vi "GeoData.vi"() -> ()   [LabVIEW 2017] (continued)
MN\tTodd County\tH1\n56331\t27153\tFreeport\tMN\tTodd County\tH1\n56378\t27153\tSauk centre\tMN\tTodd County\tH1\n56318\t27153\tBurtrum\tMN\tTodd County\tH1\n56440\t27153\tClarissa\tMN\tTodd County\tH1\n56482\t27153\tWadena\tMN\tTodd County\tH1\n56466\t27153\tMotley\tMN\tTodd County\tH1\n56446\t27153\tEagle bend\tMN\tTodd County\tH1\n56475\t27153\tRandall\tMN\tTodd County\tH1\n56389\t27153\tWest union\tMN\tTodd County\tH1\n56434\t27153\tAldrich\tMN\tTodd County\tH1\n56382\t27153\tSwanville\tMN\tTodd County\tH1\n56219\t27155\tBrowns valley\tMN\tTraverse County\tH1\n56236\t27155\tDumont\tMN\tTraverse County\tH1\n56274\t27155\tNorcross\tMN\tTraverse County\tH1\n56565\t27155\tNashua\tMN\tTraverse County\tH1\n56296\t27155\tWheaton\tMN\tTraverse County\tH1\n56211\t27155\tBeardsley\tMN\tTraverse County\tH1\n56248\t27155\tHerman\tMN\tTraverse County\tH1\n56240\t27155\tGraceville\tMN\tTraverse County\tH1\n56583\t27155\tTintah\tMN\tTraverse County\tH1\n56522\t27155\tCampbell\tMN\tTraverse County\tH1\n56221\t27155\tChokio\tMN\tTraverse County\tH1\n55906\t27157\tRochester\tMN\tWabasha County\tH1\n55960\t27157\tOronoco\tMN\tWabasha County\tH1\n55957\t27157\tMillville\tMN\tWabasha County\tH1\n55041\t27157\tLake city\tMN\tWabasha County\tH1\n55991\t27157\tZumbro falls\tMN\tWabasha County\tH1\n55027\t27157\tGoodhue\tMN\tWabasha County\tH1\n55932\t27157\tElgin\tMN\tWabasha County\tH1\n55956\t27157\tMazeppa\tMN\tWabasha County\tH1\n55910\t27157\tAltura\tMN\tWabasha County\tH1\n55945\t27157\tKellogg\tMN\tWabasha County\tH1\n55964\t27157\tPlainview\tMN\tWabasha County\tH1\n55968\t27157\tReads landing\tMN\tWabasha County\tH1\n55981\t27157\tWabasha\tMN\tWabasha County\tH1\n56481\t27159\tVerndale\tMN\tWadena County\tH1\n56464\t27159\tMenahga\tMN\tWadena County\tH1\n56470\t27159\tPark rapids\tMN\tWadena County\tH1\n56479\t27159\tStaples\tMN\tWadena County\tH1\n56477\t27159\tSebeka\tMN\tWadena County\tH1\n56482\t27159\tWadena\tMN\tWadena County\tH1\n56434\t27159\tAldrich\tMN\tWadena County\tH1\n56096\t27161\tWaterville\tMN\tWaseca County\tH1\n56068\t27161\tMinnesota lake\tMN\tWaseca County\tH1\n56078\t27161\tPemberton\tMN\tWaseca County\tH1\n56091\t27161\tWaldorf\tMN\tWaseca County\tH1\n56026\t27161\tEllendale\tMN\tWaseca County\tH1\n56063\t27161\tMadison lake\tMN\tWaseca County\tH1\n56093\t27161\tWaseca\tMN\tWaseca County\tH1\n56072\t27161\tNew richland\tMN\tWaseca County\tH1\n56042\t27161\tHartland\tMN\tWaseca County\tH1\n56065\t27161\tMapleton\tMN\tWaseca County\tH1\n56028\t27161\tElysian\tMN\tWaseca County\tH1\n56048\t27161\tJanesville\tMN\tWaseca County\tH1\n56097\t27161\tWells\tMN\tWaseca County\tH1\n55052\t27161\tMorristown\tMN\tWaseca County\tH1\n55071\t27163\tSaint paul park\tMN\tWashington County\tH1\n55016\t27163\tCottage grove\tMN\tWashington County\tH1\n55001\t27163\tAfton\tMN\tWashington County\tH1\n55042\t27163\tLake elmo\tMN\tWashington County\tH1\n55033\t27163\tHastings\tMN\tWashington County\tH1\n55013\t27163\tChisago city\tMN\tWashington County\tH1\n55043\t27163\tLakeland\tMN\tWashington County\tH1\n55055\t27163\tNewport\tMN\tWashington County\tH1\n55047\t27163\tMarine on saint croix\tMN\tWashington County\tH1\n55119\t27163\tSaint paul\tMN\tWashington County\tH1\n55025\t27163\tForest lake\tMN\tWashington County\tH1\n55073\t27163\tScandia\tMN\tWashington County\tH1\n55109\t27163\tSaint paul\tMN\tWashington County\tH1\n55125\t27163\tSaint paul\tMN\tWashington County\tH1\n55038\t27163\tHugo\tMN\tWashington County\tH1\n55082\t27163\tStillwater\tMN\tWashington County\tH1\n55115\t27163\tSaint paul\tMN\tWashington County\tH1\n55083\t27163\tStillwater\tMN\tWashington County\tH1\n55003\t27163\tBayport\tMN\tWashington County\tH1\n55110\t27163\tSaint paul\tMN\tWashington County\tH1\n55128\t27163\tSaint paul\tMN\tWashington County\tH1\n55129\t27163\tSaint paul\tMN\tWashington County\tH1\n55090\t27163\tWillernie\tMN\tWashington County\tH1\n56159\t27165\tMountain lake\tMN\tWatonwan County\tH1\n56162\t27165\tOrmsby\tMN\tWatonwan County\tH1\n56160\t27165\tOdin\tMN\tWatonwan County\tH1\n56081\t27165\tSaint james\tMN\tWatonwan County\tH1\n56022\t27165\tDarfur\tMN\tWatonwan County\tH1\n56056\t27165\tLa salle\tMN\tWatonwan County\tH1\n56062\t27165\tMadelia\tMN\tWatonwan County\tH1\n56041\t27165\tHanska\tMN\tWatonwan County\tH1\n56019\t27165\tComfrey\tMN\tWatonwan County\tH1\n56120\t27165\tButterfield\tMN\tWatonwan County\tH1\n56060\t27165\tLewisville\tMN\tWatonwan County\tH1\n56088\t27165\tTruman\tMN\tWatonwan County\tH1\n56565\t27167\tNashua\tMN\tWilkin County\tH1\n56520\t27167\tBreckenridge\tMN\tWilkin County\tH1\n56594\t27167\tWolverton\tMN\tWilkin County\tH1\n56543\t27167\tFoxhome\tMN\tWilkin County\tH1\n56579\t27167\tRothsay\tMN\tWilkin County\tH1\n56583\t27167\tTintah\tMN\tWilkin County\tH1\n56522\t27167\tCampbell\tMN\tWilkin County\tH1\n56514\t27167\tBarnesville\tMN\tWilkin County\tH1\n56572\t27167\tPelican rapids\tMN\tWilkin County\tH1\n56553\t27167\tKent\tMN\tWilkin County\tH1\n55952\t27169\tLewiston\tMN\tWinona County\tH1\n55987\t27169\tWinona\tMN\tWinona County\tH1\n55923\t27169\tChatfield\tMN\tWinona County\tH1\n55959\t27169\tMinnesota city\tMN\tWinona County\tH1\n55971\t27169\tRushford\tMN\tWinona County\tH1\n55962\t27169\tPeterson\tMN\tWinona County\tH1\n55972\t27169\tSaint charles\tMN\tWinona County\tH1\n55979\t27169\tUtica\tMN\tWinona County\tH1\n55947\t27169\tLa crescent\tMN\tWinona County\tH1\n55969\t27169\tRollingstone\tMN\tWinona County\tH1\n55910\t27169\tAltura\tMN\tWinona County\tH1\n55943\t27169\tHouston\tMN\tWinona County\tH1\n55964\t27169\tPlainview\tMN\tWinona County\tH1\n55925\t27169\tDakota\tMN\tWinona County\tH1\n55363\t27171\tMontrose\tMN\tWright County\tH1\n55341\t27171\tHanover\tMN\tWright County\tH1\n55327\t27171\tDayton\tMN\tWright County\tH1\n55376\t27171\tSaint michael\tMN\tWright County\tH1\n55330\t27171\tElk river\tMN\tWright County\tH1\n55313\t27171\tBuffalo\tMN\tWright County\tH1\n55321\t27171\tCokato\tMN\tWright County\tH1\n55328\t27171\tDelano\tMN\tWright County\tH1\n55362\t27171\tMonticello\tMN\tWright County\tH1\n55373\t27171\tRockford\tMN\tWright County\tH1\n55388\t27171\tWatertown\tMN\tWright County\tH1\n55358\t27171\tMaple lake\tMN\tWright County\tH1\n55382\t27171\tSouth haven\tMN\tWright County\tH1\n55381\t27171\tSilver lake\tMN\tWright County\tH1\n55374\t27171\tRogers\tMN\tWright County\tH1\n55301\t27171\tAlbertville\tMN\tWright County\tH1\n55320\t27171\tClearwater\tMN\tWright County\tH1\n55302\t27171\tAnnandale\tMN\tWright County\tH1\n55390\t27171\tWaverly\tMN\tWright County\tH1\n55349\t27171\tHoward lake\tMN\tWright County\tH1\n55325\t27171\tDassel\tMN\tWright County\tH1\n55395\t27171\tWinsted\tMN\tWright County\tH1\n56264\t27173\tMinneota\tMN\tYellow Medicine County\tH1\n56223\t27173\tClarkfield\tMN\tYellow Medicine County\tH1\n56291\t27173\tTaunton\tMN\tYellow Medicine County\tH1\n56256\t27173\tMadison\tMN\tYellow Medicine County\tH1\n56241\t27173\tGranite falls\tMN\tYellow Medicine County\tH1\n56142\t27173\tIvanhoe\tMN\tYellow Medicine County\tH1\n56220\t27173\tCanby\tMN\tYellow Medicine County\tH1\n56265\t27173\tMontevideo\tMN\tYellow Medicine County\tH1\n56292\t27173\tVesta\tMN\tYellow Medicine County\tH1\n56214\t27173\tBelview\tMN\tYellow Medicine County\tH1\n56297\t27173\tWood lake\tMN\tYellow Medicine County\tH1\n56218\t27173\tBoyd\tMN\tYellow Medicine County\tH1\n56229\t27173\tCottonwood\tMN\tYellow Medicine County\tH1\n56237\t27173\tEcho\tMN\tYellow Medicine County\tH1\n56245\t27173\tHanley falls\tMN\tYellow Medicine County\tH1\n56280\t27173\tPorter\tMN\tYellow Medicine County\tH1\n39121\t28001\tNatchez\tMS\tAdams County\tH1\n39661\t28001\tRoxie\tMS\tAdams County\tH1\n39122\t28001\tNatchez\tMS\tAdams County\tH1\n39190\t28001\tWashington\tMS\tAdams County\tH1\n39165\t28001\tSibley\tMS\tAdams County\tH1\n39120\t28001\tNatchez\tMS\tAdams County\tH1\n38846\t28003\tGlen\tMS\tAlcorn County\tH1\n38683\t28003\tWalnut\tMS\tAlcorn County\tH1\n38833\t28003\tBurnsville\tMS\tAlcorn County\tH1\n38865\t28003\tRienzi\tMS\tAlcorn County\tH1\n38835\t28003\tCorinth\tMS\tAlcorn County\tH1\n38834\t28003\tCorinth\tMS\tAlcorn County\tH1\n39638\t28005\tGloster\tMS\tAmite County\tH1\n39652\t28005\tMagnolia\tMS\tAmite County\tH1\n39633\t28005\tCrosby\tMS\tAmite County\tH1\n39645\t28005\tLiberty\tMS\tAmite County\tH1\n39631\t28005\tCentreville\tMS\tAmite County\tH1\n39666\t28005\tSummit\tMS\tAmite County\tH1\n39657\t28005\tOsyka\tMS\tAmite County\tH1\n39664\t28005\tSmithdale\tMS\tAmite County\tH1\n39653\t28005\tMeadville\tMS\tAmite County\tH1\n39051\t28007\tCarthage\tMS\tAttala County\tH1\n39192\t28007\tWest\tMS\tAttala County\tH1\n39090\t28007\tKosciusko\tMS\tAttala County\tH1\n39079\t28007\tGoodman\tMS\tAttala County\tH1\n39772\t28007\tWeir\tMS\tAttala County\tH1\n39108\t28007\tMc cool\tMS\tAttala County\tH1\n39160\t28007\tSallis\tMS\tAttala County\tH1\n39067\t28007\tEthel\tMS\tAttala County\tH1\n39176\t28007\tVaiden\tMS\tAttala County\tH1\n38635\t28009\tHolly springs\tMS\tBenton County\tH1\n38603\t28009\tAshland\tMS\tBenton County\tH1\n38629\t28009\tFalkner\tMS\tBenton County\tH1\n38683\t28009\tWalnut\tMS\tBenton County\tH1\n38650\t28009\tMyrtle\tMS\tBenton County\tH1\n38610\t28009\tBlue mountain\tMS\tBenton County\tH1\n38633\t28009\tHickory flat\tMS\tBenton County\tH1\n38647\t28009\tMichigan city\tMS\tBenton County\tH1\n38642\t28009\tLamar\tMS\tBenton County\tH1\n38663\t28009\tRipley\tMS\tBenton County\tH1\n38659\t28009\tPotts camp\tMS\tBenton County\tH1\n38769\t28011\tRosedale\tMS\tBolivar County\tH1\n38746\t28011\tGunnison\tMS\tBolivar County\tH1\n38781\t28011\tWinstonville\tMS\tBolivar County\tH1\n38733\t28011\tCleveland\tMS\tBolivar County\tH1\n38762\t28011\tMound bayou\tMS\tBolivar County\tH1\n38720\t28011\tAlligator\tMS\tBolivar County\tH1\n38764\t28011\tPace\tMS\tBolivar County\tH1\n38740\t28011\tDuncan\tMS\tBolivar County\tH1\n38772\t28011\tScott\tMS\tBolivar County\tH1\n38726\t28011\tBeulah\tMS\tBolivar County\tH1\n38759\t28011\tMerigold\tMS\tBolivar County\tH1\n38774\t28011\tShelby\tMS\tBolivar County\tH1\n38730\t28011\tBoyle\tMS\tBolivar County\tH1\n38614\t28011\tClarksdale\tMS\tBolivar County\tH1\n38732\t28011\tCleveland\tMS\tBolivar County\tH1\n38703\t28011\tGreenville\tMS\tBolivar County\tH1\n38725\t28011\tBenoit\tMS\tBolivar County\tH1\n38773\t28011\tShaw\tMS\tBolivar County\tH1\n38951\t28013\tPittsboro\tMS\tCalhoun County\tH1\n38929\t28013\tGore springs\tMS\tCalhoun County\tH1\n38839\t28013\tDerma\tMS\tCalhoun County\tH1\n38851\t28013\tHouston\tMS\tCalhoun County\tH1\n38913\t28013\tBanner\tMS\tCalhoun County\tH1\n38850\t28013\tHoulka\tMS\tCalhoun County\tH1\n38864\t28013\tRandolph\tMS\tCalhoun County\tH1\n38915\t28013\tBruce\tMS\tCalhoun County\tH1\n38878\t28013\tVardaman\tMS\tCalhoun County\tH1\n38914\t28013\tBig creek\tMS\tCalhoun County\tH1\n38916\t28013\tCalhoun city\tMS\tCalhoun County\tH1\n38965\t28013\tWater valley\tMS\tCalhoun County\tH1\n38954\t28015\tSidon\tMS\tCarroll County\tH1\n39192\t28015\tWest\tMS\tCarroll County\tH1\n38943\t28015\tMc carley\tMS\tCarroll County\tH1\n38947\t28015\tNorth carrollton\tMS\tCarroll County\tH1\n38917\t28015\tCarrollton\tMS\tCarroll County\tH1\n38924\t28015\tCruger\tMS\tCarroll County\tH1\n38930\t28015\tGreenwood\tMS\tCarroll County\tH1\n38967\t28015\tWinona\tMS\tCarroll County\tH1\n38940\t28015\tHolcomb\tMS\tCarroll County\tH1\n38923\t28015\tCoila\tMS\tCarroll County\tH1\n39176\t28015\tVaiden\tMS\tCarroll County\tH1\n38868\t28017\tShannon\tMS\tChickasaw County\tH1\n38851\t28017\tHouston\tMS\tChickasaw County\tH1\n38877\t28017\tVan vleet\tMS\tChickasaw County\tH1\n38850\t28017\tHoulka\tMS\tChickasaw County\tH1\n38860\t28017\tOkolona\tMS\tChickasaw County\tH1\n38878\t28017\tVardaman\tMS\tChickasaw County\tH1\n39756\t28017\tPrairie\tMS\tChickasaw County\tH1\n39730\t28017\tAberdeen\tMS\tChickasaw County\tH1\n39751\t28017\tMantee\tMS\tChickasaw County\tH1\n39776\t28017\tWoodland\tMS\tChickasaw County\tH1\n38875\t28017\tTrebloc\tMS\tChickasaw County\tH1\n39752\t28019\tMathiston\tMS\tChoctaw County\tH1\n39744\t28019\tEupora\tMS\tChoctaw County\tH1\n39767\t28019\tStewart\tMS\tChoctaw County\tH1\n39772\t28019\tWeir\tMS\tChoctaw County\tH1\n39108\t28019\tMc cool\tMS\tChoctaw County\tH1\n39745\t28019\tFrench camp\tMS\tChoctaw County\tH1\n39750\t28019\tMaben\tMS\tChoctaw County\tH1\n39735\t28019\tAckerman\tMS\tChoctaw County\tH1\n39769\t28019\tSturgis\tMS\tChoctaw County\tH1\n39144\t28021\tPattison\tMS\tClaiborne County\tH1\n39096\t28021\tLorman\tMS\tClaiborne County\tH1\n39150\t28021\tPort gibson\tMS\tClaiborne County\tH1\n39175\t28021\tUtica\tMS\tClaiborne County\tH1\n39086\t28021\tHermanville\tMS\tClaiborne County\tH1\n39363\t28023\tStonewall\tMS\tClarke County\tH1\n39307\t28023\tMeridian\tMS\tClarke County\tH1\n39360\t28023\tShubuta\tMS\tClarke County\tH1\n39367\t28023\tWaynesboro\tMS\tClarke County\tH1\n39439\t28023\tHeidelberg\tMS\tClarke County\tH1\n39355\t28023\tQuitman\tMS\tClarke County\tH1\n39366\t28023\tVossburg\tMS\tClarke County\tH1\n39347\t28023\tPachuta\tMS\tClarke County\tH1\n39301\t28023\tMeridian\tMS\tClarke County\tH1\n39330\t28023\tEnterprise\tMS\tClarke County\tH1\n39741\t28025\tCedarbluff\tMS\tClay County\tH1\n39773\t28025\tWest point\tMS\tClay County\tH1\n39755\t28025\tPheba\tMS\tClay County\tH1\n38860\t28025\tOkolona\tMS\tClay County\tH1\n39759\t28025\tStarkville\tMS\tClay County\tH1\n39756\t28025\tPrairie\tMS\tClay County\tH1\n39751\t28025\tMantee\tMS\tClay County\tH1\n39750\t28025\tMaben\tMS\tClay County\tH1\n39776\t28025\tWoodland\tMS\tClay County\tH1\n38626\t28027\tDundee\tMS\tCoahoma County\tH1\n38720\t28027\tAlligator\tMS\tCoahoma County\tH1\n38767\t28027\tRena lara\tMS\tCoahoma County\tH1\n38631\t28027\tFriars point\tMS\tCoahoma County\tH1\n38643\t28027\tLambert\tMS\tCoahoma County\tH1\n38963\t28027\tTutwiler\tMS\tCoahoma County\tH1\n38614\t28027\tClarksdale\tMS\tCoahoma County\tH1\n38617\t28027\tCoahoma\tMS\tCoahoma County\tH1\n38639\t28027\tJonestown\tMS\tCoahoma County\tH1\n38645\t28027\tLyon\tMS\tCoahoma County\tH1\n38739\t28027\tDublin\tMS\tCoahoma County\tH1\n38644\t28027\tLula\tMS\tCoahoma County\tH1\n39191\t28029\tWesson\tMS\tCopiah County\tH1\n39170\t28029\tTerry\tMS\tCopiah County\tH1\n39077\t28029\tGallman\tMS\tCopiah County\tH1\n39144\t28029\tPattison\tMS\tCopiah County\tH1\n39175\t28029\tUtica\tMS\tCopiah County\tH1\n39654\t28029\tMonticello\tMS\tCopiah County\tH1\n39083\t28029\tHazlehurst\tMS\tCopiah County\tH1\n39078\t28029\tGeorgetown\tMS\tCopiah County\tH1\n39059\t28029\tCrystal springs\tMS\tCopiah County\tH1\n39086\t28029\tHermanville\tMS\tCopiah County\tH1\n39668\t28029\tUnion church\tMS\tCopiah County\tH1\n39119\t28031\tMount olive\tMS\tCovington County\tH1\n39401\t28031\tHattiesburg\tMS\tCovington County\tH1\n39168\t28031\tTaylorsville\tMS\tCovington County\tH1\n39402\t28031\tHattiesburg\tMS\tCovington County\tH1\n39428\t28031\tCollins\tMS\tCovington County\tH1\n39479\t28031\tSeminary\tMS\tCovington County\tH1\n39474\t28031\tPrentiss\tMS\tCovington County\tH1\n39482\t28031\tSumrall\tMS\tCovington County\tH1\n39437\t28031\tEllisville\tMS\tCovington County\tH1\n38686\t28033\tWalls\tMS\tDeSoto County\tH1\n38632\t28033\tHernando\tMS\tDeSoto County\tH1\n38637\t28033\tHorn lake\tMS\tDeSoto County\tH1\n38671\t28033\tSouthaven\tMS\tDeSoto County\tH1\n38680\t28033\tWalls\tMS\tDeSoto County\tH1\n38641\t28033\tLake cormorant\tMS\tDeSoto County\tH1\n38611\t28033\tByhalia\tMS\tDeSoto County\tH1\n38618\t28033\tColdwater\tMS\tDeSoto County\tH1\n38654\t28033\tOlive branch\tMS\tDeSoto County\tH1\n38651\t28033\tNesbit\tMS\tDeSoto County\tH1\n38672\t28033\tSouthaven\tMS\tDeSoto County\tH1\n39403\t28035\tHattiesburg\tMS\tForrest County\tH1\n39465\t28035\tPetal\tMS\tForrest County\tH1\n39577\t28035\tWiggins\tMS\tForrest County\tH1\n39407\t28035\tHattiesburg\tMS\tForrest County\tH1\n39401\t28035\tHattiesburg\tMS\tForrest County\tH1\n39425\t28035\tBrooklyn\tMS\tForrest County\tH1\n39402\t28035\tHattiesburg\tMS\tForrest County\tH1\n39455\t28035\tLumberton\tMS\tForrest County\tH1\n39404\t28035\tHattiesburg\tMS\tForrest County\tH1\n39406\t28035\tHattiesburg\tMS\tForrest County\tH1\n39437\t28035\tEllisville\tMS\tForrest County\tH1\n39475\t28035\tPurvis\tMS\tForrest County\tH1\n39647\t28037\tMc call creek\tMS\tFranklin County\tH1\n39661\t28037\tRoxie\tMS\tFranklin County\tH1\n39601\t28037\tBrookhaven\tMS\tFranklin County\tH1\n39664\t28037\tSmithdale\tMS\tFranklin County\tH1\n39653\t28037\tMeadville\tMS\tFranklin County\tH1\n39668\t28037\tUnion church\tMS\tFranklin County\tH1\n39630\t28037\tBude\tMS\tFranklin County\tH1\n39456\t28039\tMc lain\tMS\tGeorge County\tH1\n39452\t28039\tLucedale\tMS\tGeorge County\tH1\n39573\t28039\tPerkinston\tMS\tGeorge County\tH1\n39456\t28041\tMc lain\tMS\tGreene County\tH1\n39362\t28041\tState line\tMS\tGreene County\tH1\n39476\t28041\tRichton\tMS\tGreene County\tH1\n39423\t28041\tBeaumont\tMS\tGreene County\tH1\n39451\t28041\tLeakesville\tMS\tGreene County\tH1\n39452\t28041\tLucedale\tMS\tGreene County\tH1\n39461\t28041\tNeely\tMS\tGreene County\tH1\n38925\t28043\tDuck hill\tMS\tGrenada County\tH1\n38929\t28043\tGore springs\tMS\tGrenada County\tH1\n39744\t28043\tEupora\tMS\tGrenada County\tH1\n38922\t28043\tCoffeeville\tMS\tGrenada County\tH1\n38920\t28043\tCascilla\tMS\tGrenada County\tH1\n38953\t28043\tScobey\tMS\tGrenada County\tH1\n38914\t28043\tBig creek\tMS\tGrenada County\tH1\n38960\t28043\tTie plant\tMS\tGrenada County\tH1\n38901\t28043\tGrenada\tMS\tGrenada County\tH1\n38940\t28043\tHolcomb\tMS\tGrenada County\tH1\n38961\t28043\tTillatoba\tMS\tGrenada County\tH1\n39556\t28045\tKiln\tMS\tHancock County\tH1\n39426\t28045\tCarriere\tMS\tHancock County\tH1\n39466\t28045\tPicayune\tMS\tHancock County\tH1\n39470\t28045\tPoplarville\tMS\tHancock County\tH1\n39520\t28045\tBay saint louis\tMS\tHancock County\tH1\n39572\t28045\tPearlington\tMS\tHancock County\tH1\n39558\t28045\tLakeshore\tMS\tHancock County\tH1\n39576\t28045\tWaveland\tMS\tHancock County\tH1\n39571\t28045\tPass christian\tMS\tHancock County\tH1\n39525\t28045\tDiamondhead\tMS\tHancock County\tH1\n39573\t28045\tPerkinston\tMS\tHancock County\tH1\n39529\t28045\tStennis space center\tMS\tHancock County\tH1\n39522\t28045\tStennis space center\tMS\tHancock County\tH1\n39560\t28047\tLong beach\tMS\tHarrison County\tH1\n39507\t28047\tGulfport\tMS\tHarrison County\tH1\n39530\t28047\tBiloxi\tMS\tHarrison County\tH1\n39501\t28047\tGulfport\tMS\tHarrison County\tH1\n39574\t28047\tSaucier\tMS\tHarrison County\tH1\n39534\t28047\tBiloxi\tMS\tHarrison County\tH1\n39565\t28047\tVancleave\tMS\tHarrison County\tH1\n39532\t28047\tBiloxi\tMS\tHarrison County\tH1\n39540\t28047\tDiberville\tMS\tHarrison County\tH1\n39535\t28047\tBiloxi\tMS\tHarrison County\tH1\n39503\t28047\tGulfport\tMS\tHarrison County\tH1\n39531\t28047\tBiloxi\tMS\tHarrison County\tH1\n39506\t28047\tGulfport\tMS\tHarrison County\tH1\n39533\t28047\tBiloxi\tMS\tHarrison County\tH1\n39571\t28047\tPass christian\tMS\tHarrison County\tH1\n39573\t28047\tPerkinston\tMS\tHarrison County\tH1\n39505\t28047\tGulfport\tMS\tHarrison County\tH1\n39502\t28047\tGulfport\tMS\tHarrison County\tH1\n39066\t28049\tEdwards\tMS\tHinds County\tH1\n39201\t28049\tJackson\tMS\tHinds County\tH1\n39205\t28049\tJackson\tMS\tHinds County\tH1\n39217\t28049\tJackson\tMS\tHinds County\tH1\n39210\t28049\tJackson\tMS\tHinds County\tH1\n39286\t28049\tJackson\tMS\tHinds County\tH1\n39211\t28049\tJackson\tMS\tHinds County\tH1\n39206\t28049\tJackson\tMS\tHinds County\tH1\n39272\t28049\tByram\tMS\tHinds County\tH1\n39170\t28049\tTerry\tMS\tHinds County\tH1\n39203\t28049\tJackson\tMS\tHinds County\tH1\n39216\t28049\tJackson\tMS\tHinds County\tH1\n39215\t28049\tJackson\tMS\tHinds County\tH1\n39283\t28049\tJackson\tMS\tHinds County\tH1\n39212\t28049\tJackson\tMS\tHinds County\tH1\n39204\t28049\tJackson\tMS\tHinds County\tH1\n39175\t28049\tUtica\tMS\tHinds County\tH1\n39207\t28049\tJackson\tMS\tHinds County\tH1\n39296\t28049\tJackson\tMS\tHinds County\tH1\n39059\t28049\tCrystal springs\tMS\tHinds County\tH1\n39060\t28049\tClinton\tMS\tHinds County\tH1\n39202\t28049\tJackson\tMS\tHinds County\tH1\n39209\t28049\tJackson\tMS\tHinds County\tH1\n39213\t28049\tJackson\tMS\tHinds County\tH1\n39058\t28049\tClinton\tMS\tHinds County\tH1\n39086\t28049\tHermanville\tMS\tHinds County\tH1\n39232\t28049\tFlowood\tMS\tHinds County\tH1\n39174\t28049\tTougaloo\tMS\tHinds County\tH1\n39269\t28049\tJackson\tMS\tHinds County\tH1\n39056\t28049\tClinton\tMS\tHinds County\tH1\n39041\t28049\tBolton\tMS\tHinds County\tH1\n39154\t28049\tRaymond\tMS\tHinds County\tH1\n39208\t28049\tPearl\tMS\tHinds County\tH1\n39236\t28049\tJackson\tMS\tHinds County\tH1\n39284\t28049\tJackson\tMS\tHinds County\tH1\n39225\t28049\tJackson\tMS\tHinds County\tH1\n38954\t28051\tSidon\tMS\tHolmes County\tH1\n39192\t28051\tWest\tMS\tHolmes County\tH1\n39146\t28051\tPickens\tMS\tHolmes County\tH1\n39038\t28051\tBelzoni\tMS\tHolmes County\tH1\n39079\t28051\tGoodman\tMS\tHolmes County\tH1\n39169\t28051\tTchula\tMS\tHolmes County\tH1\n38924\t28051\tCruger\tMS\tHolmes County\tH1\n39095\t28051\tLexington\tMS\tHolmes County\tH1\n39063\t28051\tDurant\tMS\tHolmes County\tH1\n38753\t28053\tInverness\tMS\tHumphreys County\tH1\n38754\t28053\tIsola\tMS\tHumphreys County\tH1\n39194\t28053\tYazoo city\tMS\tHumphreys County\tH1\n39115\t28053\tMidnight\tMS\tHumphreys County\tH1\n39166\t28053\tSilver city\tMS\tHumphreys County\tH1\n39038\t28053\tBelzoni\tMS\tHumphreys County\tH1\n39097\t28053\tLouise\tMS\tHumphreys County\tH1\n39159\t28055\tRolling fork\tMS\tIssaquena County\tH1\n39113\t28055\tMayersville\tMS\tIssaquena County\tH1\n39183\t28055\tVicksburg\tMS\tIssaquena County\tH1\n38744\t28055\tGlen allan\tMS\tIssaquena County\tH1\n39177\t28055\tValley park\tMS\tIssaquena County\tH1\n38745\t28055\tGrace\tMS\tIssaquena County\tH1\n38849\t28057\tGuntown\tMS\tItawamba County\tH1\n38848\t28057\tGreenwood springs\tMS\tItawamba County\tH1\n38843\t28057\tFulton\tMS\tItawamba County\tH1\n38857\t28057\tMooreville\tMS\tItawamba County\tH1\n38804\t28057\tTupelo\tMS\tItawamba County\tH1\n38847\t28057\tGolden\tMS\tItawamba County\tH1\n38855\t28057\tMantachie\tMS\tItawamba County\tH1\n38824\t28057\tBaldwyn\tMS\tItawamba County\tH1\n38876\t28057\tTremont\tMS\tItawamba County\tH1\n38858\t28057\tNettleton\tMS\tItawamba County\tH1\n38856\t28057\tMarietta\tMS\tItawamba County\tH1\n38870\t28057\tSmithville\tMS\tItawamba County\tH1\n39553\t28059\tGautier\tMS\tJackson County\tH1\n39552\t28059\tEscatawpa\tMS\tJackson County\tH1\n39562\t28059\tMoss point\tMS\tJackson County\tH1\n39563\t28059\tMoss point\tMS\tJackson County\tH1\n39567\t28059\tPascagoula\tMS\tJackson County\tH1\n39595\t28059\tPascagoula\tMS\tJackson County\tH1\n39566\t28059\tOcean springs\tMS\tJackson County\tH1\n39452\t28059\tLucedale\tMS\tJackson County\tH1\n39565\t28059\tVancleave\tMS\tJackson County\tH1\n39532\t28059\tBiloxi\tMS\tJackson County\tH1\n39581\t28059\tPascagoula\tMS\tJackson County\tH1\n39569\t28059\tPascagoula\tMS\tJackson County\tH1\n39564\t28059\tOcean springs\tMS\tJackson County\tH1\n39573\t28059\tPerkinston\tMS\tJackson County\tH1\n39555\t28059\tHurley\tMS\tJackson County\tH1\n39443\t28061\tLaurel\tMS\tJasper County\tH1\n39480\t28061\tSoso\tMS\tJasper County\tH1\n39153\t28061\tRaleigh\tMS\tJasper County\tH1\n39336\t28061\tLawrence\tMS\tJasper County\tH1\n39168\t28061\tTaylorsville\tMS\tJasper County\tH1\n39332\t28061\tHickory\tMS\tJasper County\tH1\n39439\t28061\tHeidelberg\tMS\tJasper County\tH1\n39460\t28061\tMoss\tMS\tJasper County\tH1\n39422\t28061\tBay springs\tMS\tJasper County\tH1\n39366\t28061\tVossburg\tMS\tJasper County\tH1\n39348\t28061\tPaulding\tMS\tJasper County\tH1\n39338\t28061\tLouin\tMS\tJasper County\tH1\n39347\t28061\tPachuta\tMS\tJasper County\tH1\n39356\t28061\tRose hill\tMS\tJasper County\tH1\n39345\t28061\tNewton\tMS\tJasper County\tH1\n39481\t28061\tStringer\tMS\tJasper County\tH1\n39330\t28061\tEnterprise\tMS\tJasper County\tH1\n39069\t28063\tFayette\tMS\tJefferson County\tH1\n39661\t28063\tRoxie\tMS\tJefferson County\tH1\n39144\t28063\tPattison\tMS\tJefferson County\tH1\n39096\t28063\tLorman\tMS\tJefferson County\tH1\n39120\t28063\tNatchez\tMS\tJefferson County\tH1\n39653\t28063\tMeadville\tMS\tJefferson County\tH1\n39668\t28063\tUnion church\tMS\tJefferson County\tH1\n39119\t28065\tMount olive\tMS\tJefferson Davis County\tH1\n39421\t28065\tBassfield\tMS\tJefferson Davis County\tH1\n39140\t28065\tNewhebron\tMS\tJefferson Davis County\tH1\n39663\t28065\tSilver creek\tMS\tJefferson Davis County\tH1\n39149\t28065\tPinola\tMS\tJefferson Davis County\tH1\n39427\t28065\tCarson\tMS\tJefferson Davis County\tH1\n39429\t28065\tColumbia\tMS\tJefferson Davis County\tH1\n39474\t28065\tPrentiss\tMS\tJefferson Davis County\tH1\n39482\t28065\tSumrall\tMS\tJefferson Davis County\tH1\n39656\t28065\tOak vale\tMS\tJefferson Davis County\tH1\n39443\t28067\tLaurel\tMS\tJones County\tH1\n39480\t28067\tSoso\tMS\tJones County\tH1\n39477\t28067\tSandersville\tMS\tJones County\tH1\n39465\t28067\tPetal\tMS\tJones County\tH1\n39401\t28067\tHattiesburg\tMS\tJones County\tH1\n39168\t28067\tTaylorsville\tMS\tJones County\tH1\n39476\t28067\tRichton\tMS\tJones County\tH1\n39439\t28067\tHeidelberg\tMS\tJones County\tH1\n39464\t28067\tOvett\tMS\tJones County\tH1\n39479\t28067\tSeminary\tMS\tJones County\tH1\n39459\t28067\tMoselle\tMS\tJones County\tH1\n39440\t28067\tLaurel\tMS\tJones County\tH1\n39436\t28067\tEastabuchie\tMS\tJones County\tH1\n39437\t28067\tEllisville\tMS\tJones County\tH1\n39320\t28069\tBailey\tMS\tKemper County\tH1\n39361\t28069\tShuqualak\tMS\tKemper County\tH1\n39350\t28069\tPhiladelphia\tMS\tKemper County\tH1\n39335\t28069\tLauderdale\tMS\tKemper County\tH1\n39325\t28069\tCollinsville\tMS\tKemper County\tH1\n39328\t28069\tDe kalb\tMS\tKemper County\tH1\n39352\t28069\tPorterville\tMS\tKemper County\tH1\n39354\t28069\tPreston\tMS\tKemper County\tH1\n39358\t28069\tScooba\tMS\tKemper County\tH1\n39341\t28069\tMacon\tMS\tKemper County\tH1\n39326\t28069\tDaleville\tMS\tKemper County\tH1\n38619\t28071\tComo\tMS\tLafayette County\tH1\n38685\t28071\tWaterford\tMS\tLafayette County\tH1\n38913\t28071\tBanner\tMS\tLafayette County\tH1\n38677\t28071\tUniversity\tMS\tLafayette County\tH1\n38627\t28071\tEtta\tMS\tLafayette County\tH1\n38601\t28071\tAbbeville\tMS\tLafayette County\tH1\n38673\t28071\tTaylor\tMS\tLafayette County\tH1\n38655\t28071\tOxford\tMS\tLafayette County\tH1\n38915\t28071\tBruce\tMS\tLafayette County\tH1\n38606\t28071\tBatesville\tMS\tLafayette County\tH1\n38871\t28071\tThaxton\tMS\tLafayette County\tH1\n38863\t28071\tPontotoc\tMS\tLafayette County\tH1\n38965\t28071\tWater valley\tMS\tLafayette County\tH1\n38949\t28071\tParis\tMS\tLafayette County\tH1\n39401\t28073\tHattiesburg\tMS\tLamar County\tH1\n39402\t28073\tHattiesburg\tMS\tLamar County\tH1\n39455\t28073\tLumberton\tMS\tLamar County\tH1\n39429\t28073\tColumbia\tMS\tLamar County\tH1\n39482\t28073\tSumrall\tMS\tLamar County\tH1\n39475\t28073\tPurvis\tMS\tLamar County\tH1\n39320\t28075\tBailey\tMS\tLauderdale County\tH1\n39309\t28075\tMeridian\tMS\tLauderdale County\tH1\n39305\t28075\tMeridian\tMS\tLauderdale County\tH1\n39307\t28075\tMeridian\tMS\tLauderdale County\tH1\n39335\t28075\tLauderdale\tMS\tLauderdale County\tH1\n39325\t28075\tCollinsville\tMS\tLauderdale County\tH1\n39342\t28075\tMarion\tMS\tLauderdale County\tH1\n39302\t28075\tMeridian\tMS\tLauderdale County\tH1\n39323\t28075\tChunky\tMS\tLauderdale County\tH1\n39364\t28075\tToomsuba\tMS\tLauderdale County\tH1\n39301\t28075\tMeridian\tMS\tLauderdale County\tH1\n39330\t28075\tEnterprise\tMS\tLauderdale County\tH1\n39326\t28075\tDaleville\tMS\tLauderdale County\tH1\n39191\t28077\tWesson\tMS\tLawrence County\tH1\n39140\t28077\tNewhebron\tMS\tLawrence County\tH1\n39641\t28077\tJayess\tMS\tLawrence County\tH1\n39654\t28077\tMonticello\tMS\tLawrence County\tH1\n39663\t28077\tSilver creek\tMS\tLawrence County\tH1\n39662\t28077\tRuth\tMS\tLawrence County\tH1\n39474\t28077\tPrentiss\tMS\tLawrence County\tH1\n39656\t28077\tOak vale\tMS\tLawrence County\tH1\n39665\t28077\tSontag\tMS\tLawrence County\tH1\n39051\t28079\tCarthage\tMS\tLeake County\tH1\n39365\t28079\tUnion\tMS\tLeake County\tH1\n39350\t28079\tPhiladelphia\tMS\tLeake County\tH1\n39171\t28079\tThomastown\tMS\tLeake County\tH1\n39109\t28079\tMadden\tMS\tLeake County\tH1\n39090\t28079\tKosciusko\tMS\tLeake County\tH1\n39160\t28079\tSallis\tMS\tLeake County\tH1\n39189\t28079\tWalnut grove\tMS\tLeake County\tH1\n39094\t28079\tLena\tMS\tLeake County\tH1\n38849\t28081\tGuntown\tMS\tLee County\tH1\n38866\t28081\tSaltillo\tMS\tLee County\tH1\n38868\t28081\tShannon\tMS\tLee County\tH1\n38828\t28081\tBlue springs\tMS\tLee County\tH1\n38801\t28081\tTupelo\tMS\tLee County\tH1\n38843\t28081\tFulton\tMS\tLee County\tH1\n38857\t28081\tMooreville\tMS\tLee County\tH1\n38804\t28081\tTupelo\tMS\tLee County\tH1\n38860\t28081\tOkolona\tMS\tLee County\tH1\n38826\t28081\tBelden\tMS\tLee County\tH1\n38855\t28081\tMantachie\tMS\tLee County\tH1\n38862\t28081\tPlantersville\tMS\tLee County\tH1\n38824\t28081\tBaldwyn\tMS\tLee County\tH1\n38858\t28081\tNettleton\tMS\tLee County\tH1\n38802\t28081\tTupelo\tMS\tLee County\tH1\n38803\t28081\tTupelo\tMS\tLee County\tH1\n38879\t28081\tVerona\tMS\tLee County\tH1\n38954\t28083\tSidon\tMS\tLeflore County\tH1\n38736\t28083\tDoddsville\tMS\tLeflore County\tH1\n38952\t28083\tSchlater\tMS\tLeflore County\tH1\n38959\t28083\tSwiftown\tMS\tLeflore County\tH1\n38761\t28083\tMoorhead\tMS\tLeflore County\tH1\n39038\t28083\tBelzoni\tMS\tLeflore County\tH1\n38924\t28083\tCruger\tMS\tLeflore County\tH1\n38950\t28083\tPhilipp\tMS\tLeflore County\tH1\n38944\t28083\tMinter city\tMS\tLeflore County\tH1\n38946\t28083\tMorgan city\tMS\tLeflore County\tH1\n38930\t28083\tGreenwood\tMS\tLeflore County\tH1\n38737\t28083\tDrew\tMS\tLeflore County\tH1\n38941\t28083\tItta bena\tMS\tLeflore County\tH1\n39647\t28085\tMc call creek\tMS\tLincoln County\tH1\n39191\t28085\tWesson\tMS\tLincoln County\tH1\n39629\t28085\tBogue chitto\tMS\tLincoln County\tH1\n39641\t28085\tJayess\tMS\tLincoln County\tH1\n39654\t28085\tMonticello\tMS\tLincoln County\tH1\n39603\t28085\tBrookhaven\tMS\tLincoln County\tH1\n39083\t28085\tHazlehurst\tMS\tLincoln County\tH1\n39602\t28085\tBrookhaven\tMS\tLincoln County\tH1\n39601\t28085\tBrookhaven\tMS\tLincoln County\tH1\n39666\t28085\tSummit\tMS\tLincoln County\tH1\n39662\t28085\tRuth\tMS\tLincoln County\tH1\n39665\t28085\tSontag\tMS\tLincoln County\tH1\n39664\t28085\tSmithdale\tMS\tLincoln County\tH1\n39668\t28085\tUnion church\tMS\tLincoln County\tH1\n39705\t28087\tColumbus\tMS\tLowndes County\tH1\n39766\t28087\tSteens\tMS\tLowndes County\tH1\n39743\t28087\tCrawford\tMS\tLowndes County\tH1\n39740\t28087\tCaledonia\tMS\tLowndes County\tH1\n39753\t28087\tMayhew\tMS\tLowndes County\tH1\n39704\t28087\tColumbus\tMS\tLowndes County\tH1\n39759\t28087\tStarkville\tMS\tLowndes County\tH1\n39701\t28087\tColumbus\tMS\tLowndes County\tH1\n39710\t28087\tColumbus\tMS\tLowndes County\tH1\n39739\t28087\tBrooksville\tMS\tLowndes County\tH1\n39703\t28087\tColumbus\tMS\tLowndes County\tH1\n39736\t28087\tArtesia\tMS\tLowndes County\tH1\n39702\t28087\tColumbus\tMS\tLowndes County\tH1\n39051\t28089\tCarthage\tMS\tMadison County\tH1\n39163\t28089\tSharon\tMS\tMadison County\tH1\n39146\t28089\tPickens\tMS\tMadison County\tH1\n39046\t28089\tCanton\tMS\tMadison County\tH1\n39079\t28089\tGoodman\tMS\tMadison County\tH1\n39157\t28089\tRidgeland\tMS\tMadison County\tH1\n39130\t28089\tMadison\tMS\tMadison County\tH1\n39110\t28089\tMadison\tMS\tMadison County\tH1\n39045\t28089\tCamden\tMS\tMadison County\tH1\n39209\t28089\tJackson\tMS\tMadison County\tH1\n39213\t28089\tJackson\tMS\tMadison County\tH1\n39158\t28089\tRidgeland\tMS\tMadison County\tH1\n39041\t28089\tBolton\tMS\tMadison County\tH1\n39071\t28089\tFlora\tMS\tMadison County\tH1\n39667\t28091\tTylertown\tMS\tMarion County\tH1\n39421\t28091\tBassfield\tMS\tMarion County\tH1\n39483\t28091\tFoxworth\tMS\tMarion County\tH1\n39455\t28091\tLumberton\tMS\tMarion County\tH1\n39643\t28091\tKokomo\tMS\tMarion County\tH1\n39478\t28091\tSandy hook\tMS\tMarion County\tH1\n39429\t28091\tColumbia\tMS\tMarion County\tH1\n39482\t28091\tSumrall\tMS\tMarion County\tH1\n38635\t28093\tHolly springs\tMS\tMarshall County\tH1\n38649\t28093\tMount pleasant\tMS\tMarshall County\tH1\n38685\t28093\tWaterford\tMS\tMarshall County\tH1\n38661\t28093\tRed banks\tMS\tMarshall County\tH1\n38611\t28093\tByhalia\tMS\tMarshall County\tH1\n38642\t28093\tLamar\tMS\tMarshall County\tH1\n38679\t28093\tVictoria\tMS\tMarshall County\tH1\n38618\t28093\tColdwater\tMS\tMarshall County\tH1\n38654\t28093\tOlive branch\tMS\tMarshall County\tH1\n38659\t28093\tPotts camp\tMS\tMarshall County\tH1\n38848\t28095\tGreenwood springs\tMS\tMonroe County\tH1\n38868\t28095\tShannon\tMS\tMonroe County\tH1\n39773\t28095\tWest point\tMS\tMonroe County\tH1\n38821\t28095\tAmory\tMS\tMonroe County\tH1\n39740\t28095\tCaledonia\tMS\tMonroe County\tH1\n39746\t28095\tHamilton\tMS\tMonroe County\tH1\n38860\t28095\tOkolona\tMS\tMonroe County\tH1\n39759\t28095\tStarkville\tMS\tMonroe County\tH1\n39756\t28095\tPrairie\tMS\tMonroe County\tH1\n39730\t28095\tAberdeen\tMS\tMonroe County\tH1\n38858\t28095\tNettleton\tMS\tMonroe County\tH1\n38870\t28095\tSmithville\tMS\tMonroe County\tH1\n38844\t28095\tGattman\tMS\tMonroe County\tH1\n38825\t28095\tBecker\tMS\tMonroe County\tH1\n39747\t28097\tKilmichael\tMS\tMontgomery County\tH1\n38925\t28097\tDuck hill\tMS\tMontgomery County\tH1\n39767\t28097\tStewart\tMS\tMontgomery County\tH1\n39745\t28097\tFrench camp\tMS\tMontgomery County\tH1\n38901\t28097\tGrenada\tMS\tMontgomery County\tH1\n38967\t28097\tWinona\tMS\tMontgomery County\tH1\n39176\t28097\tVaiden\tMS\tMontgomery County\tH1\n39051\t28099\tCarthage\tMS\tNeshoba County\tH1\n39365\t28099\tUnion\tMS\tNeshoba County\tH1\n39350\t28099\tPhiladelphia\tMS\tNeshoba County\tH1\n39337\t28099\tLittle rock\tMS\tNeshoba County\tH1\n39325\t28099\tCollinsville\tMS\tNeshoba County\tH1\n39328\t28099\tDe kalb\tMS\tNeshoba County\tH1\n39354\t28099\tPreston\tMS\tNeshoba County\tH1\n39346\t28099\tNoxapater\tMS\tNeshoba County\tH1\n39365\t28101\tUnion\tMS\tNewton County\tH1\n39337\t28101\tLittle rock\tMS\tNewton County\tH1\n39336\t28101\tLawrence\tMS\tNewton County\tH1\n39332\t28101\tHickory\tMS\tNewton County\tH1\n39325\t28101\tCollinsville\tMS\tNewton County\tH1\n39092\t28101\tLake\tMS\tNewton County\tH1\n39323\t28101\tChunky\tMS\tNewton County\tH1\n39345\t28101\tNewton\tMS\tNewton County\tH1\n39057\t28101\tConehatta\tMS\tNewton County\tH1\n39327\t28101\tDecatur\tMS\tNewton County\tH1\n39330\t28101\tEnterprise\tMS\tNewton County\tH1\n39361\t28103\tShuqualak\tMS\tNoxubee County\tH1\n39743\t28103\tCrawford\tMS\tNoxubee County\tH1\n39759\t28103\tStarkville\tMS\tNoxubee County\tH1\n39354\t28103\tPreston\tMS\tNoxubee County\tH1\n39701\t28103\tColumbus\tMS\tNoxubee County\tH1\n39739\t28103\tBrooksville\tMS\tNoxubee County\tH1\n39341\t28103\tMacon\tMS\tNoxubee County\tH1\n39752\t28105\tMathiston\tMS\tOktibbeha County\tH1\n39743\t28105\tCrawford\tMS\tOktibbeha County\tH1\n39755\t28105\tPheba\tMS\tOktibbeha County\tH1\n39759\t28105\tStarkville\tMS\tOktibbeha County\tH1\n39701\t28105\tColumbus\tMS\tOktibbeha County\tH1\n39750\t28105\tMaben\tMS\tOktibbeha County\tH1\n39735\t28105\tAckerman\tMS\tOktibbeha County\tH1\n39769\t28105\tSturgis\tMS\tOktibbeha County\tH1\n39739\t28105\tBrooksville\tMS\tOktibbeha County\tH1\n39760\t28105\tStarkville\tMS\tOktibbeha County\tH1\n39762\t28105\tMississippi state\tMS\tOktibbeha County\tH1\n38927\t28107\tEnid\tMS\tPanola County\tH1\n38619\t28107\tComo\tMS\tPanola County\tH1\n38646\t28107\tMarks\tMS\tPanola County\tH1\n38668\t28107\tSenatobia\tMS\tPanola County\tH1\n38620\t28107\tCourtland\tMS\tPanola County\tH1\n38655\t28107\tOxford\tMS\tPanola County\tH1\n38643\t28107\tLambert\tMS\tPanola County\tH1\n38670\t28107\tSledge\tMS\tPanola County\tH1\n38606\t28107\tBatesville\tMS\tPanola County\tH1\n38621\t28107\tCrenshaw\tMS\tPanola County\tH1\n38666\t28107\tSardis\tMS\tPanola County\tH1\n38665\t28107\tSarah\tMS\tPanola County\tH1\n38658\t28107\tPope\tMS\tPanola County\tH1\n38965\t28107\tWater valley\tMS\tPanola County\tH1\n39426\t28109\tCarriere\tMS\tPearl River County\tH1\n39466\t28109\tPicayune\tMS\tPearl River County\tH1\n39470\t28109\tPoplarville\tMS\tPearl River County\tH1\n39455\t28109\tLumberton\tMS\tPearl River County\tH1\n39457\t28109\tMc neill\tMS\tPearl River County\tH1\n39573\t28109\tPerkinston\tMS\tPearl River County\tH1\n39463\t28109\tNicholson\tMS\tPearl River County\tH1\n39456\t28111\tMc lain\tMS\tPerry County\tH1\n39465\t28111\tPetal\tMS\tPerry County\tH1\n39577\t28111\tWiggins\tMS\tPerry County\tH1\n39425\t28111\tBrooklyn\tMS\tPerry County\tH1\n39462\t28111\tNew augusta\tMS\tPerry County\tH1\n39476\t28111\tRichton\tMS\tPerry County\tH1\n39423\t28111\tBeaumont\tMS\tPerry County\tH1\n39464\t28111\tOvett\tMS\tPerry County\tH1\n39652\t28113\tMagnolia\tMS\tPike County\tH1\n39667\t28113\tTylertown\tMS\tPike County\tH1\n39632\t28113\tChatawa\tMS\tPike County\tH1\n39629\t28113\tBogue chitto\tMS\tPike County\tH1\n39641\t28113\tJayess\tMS\tPike County\tH1\n39666\t28113\tSummit\tMS\tPike County\tH1\n39662\t28113\tRuth\tMS\tPike County\tH1\n39635\t28113\tFernwood\tMS\tPike County\tH1\n39648\t28113\tMccomb\tMS\tPike County\tH1\n39649\t28113\tMccomb\tMS\tPike County\tH1\n39657\t28113\tOsyka\tMS\tPike County\tH1\n38868\t28115\tShannon\tMS\tPontotoc County\tH1\n38652\t28115\tNew albany\tMS\tPontotoc County\tH1\n38828\t28115\tBlue springs\tMS\tPontotoc County\tH1\n38801\t28115\tTupelo\tMS\tPontotoc County\tH1\n38627\t28115\tEtta\tMS\tPontotoc County\tH1\n38804\t28115\tTupelo\tMS\tPontotoc County\tH1\n38841\t28115\tEcru\tMS\tPontotoc County\tH1\n38655\t28115\tOxford\tMS\tPontotoc County\tH1\n38850\t28115\tHoulka\tMS\tPontotoc County\tH1\n38860\t28115\tOkolona\tMS\tPontotoc County\tH1\n38826\t28115\tBelden\tMS\tPontotoc County\tH1\n38864\t28115\tRandolph\tMS\tPontotoc County\tH1\n38869\t28115\tSherman\tMS\tPontotoc County\tH1\n38874\t28115\tToccopola\tMS\tPontotoc County\tH1\n38871\t28115\tThaxton\tMS\tPontotoc County\tH1\n38863\t28115\tPontotoc\tMS\tPontotoc County\tH1\n38820\t28115\tAlgoma\tMS\tPontotoc County\tH1\n38873\t28117\tTishomingo\tMS\tPrentiss County\tH1\n38829\t28117\tBooneville\tMS\tPrentiss County\tH1\n38833\t28117\tBurnsville\tMS\tPrentiss County\tH1\n38880\t28117\tWheeler\tMS\tPrentiss County\tH1\n38824\t28117\tBaldwyn\tMS\tPrentiss County\tH1\n38865\t28117\tRienzi\tMS\tPrentiss County\tH1\n38859\t28117\tNew site\tMS\tPrentiss County\tH1\n38856\t28117\tMarietta\tMS\tPrentiss County\tH1\n38646\t28119\tMarks\tMS\tQuitman County\tH1\n38643\t28119\tLambert\tMS\tQuitman County\tH1\n38670\t28119\tSledge\tMS\tQuitman County\tH1\n38963\t28119\tTutwiler\tMS\tQuitman County\tH1\n38606\t28119\tBatesville\tMS\tQuitman County\tH1\n38621\t28119\tCrenshaw\tMS\tQuitman County\tH1\n38617\t28119\tCoahoma\tMS\tQuitman County\tH1\n38964\t28119\tVance\tMS\tQuitman County\tH1\n38645\t28119\tLyon\tMS\tQuitman County\tH1\n38622\t28119\tCrowder\tMS\tQuitman County\tH1\n38623\t28119\tDarling\tMS\tQuitman County\tH1\n39218\t28121\tRichland\tMS\tRankin County\tH1\n39042\t28121\tBrandon\tMS\tRankin County\tH1\n39272\t28121\tByram\tMS\tRankin County\tH1\n39073\t28121\tFlorence\tMS\tRankin County\tH1\n39298\t28121\tJackson\tMS\tRankin County\tH1\n39117\t28121\tMorton\tMS\tRankin County\tH1\n39167\t28121\tStar\tMS\tRankin County\tH1\n39047\t28121\tBrandon\tMS\tRankin County\tH1\n39161\t28121\tSandhill\tMS\tRankin County\tH1\n39193\t28121\tWhitfield\tMS\tRankin County\tH1\n39145\t28121\tPelahatchie\tMS\tRankin County\tH1\n39043\t28121\tBrandon\tMS\tRankin County\tH1\n39232\t28121\tFlowood\tMS\tRankin County\tH1\n39288\t28121\tPearl\tMS\tRankin County\tH1\n39094\t28121\tLena\tMS\tRankin County\tH1\n39044\t28121\tBraxton\tMS\tRankin County\tH1\n39114\t28121\tMendenhall\tMS\tRankin County\tH1\n39208\t28121\tPearl\tMS\tRankin County\tH1\n39151\t28121\tPuckett\tMS\tRankin County\tH1\n39148\t28121\tPiney woods\tMS\tRankin 
